vi "ex_getErrorSource.vi"(1 "error in (no error)":errorcluster) -> (0 "error out":errorcluster)   [LabVIEW 2017]
panel:
  in  "Localized ' in ' in message 'foo.vi in bar.vi'":string=" in "
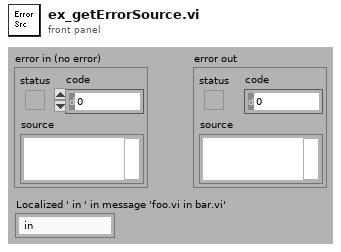
[diagram p1: front panel]
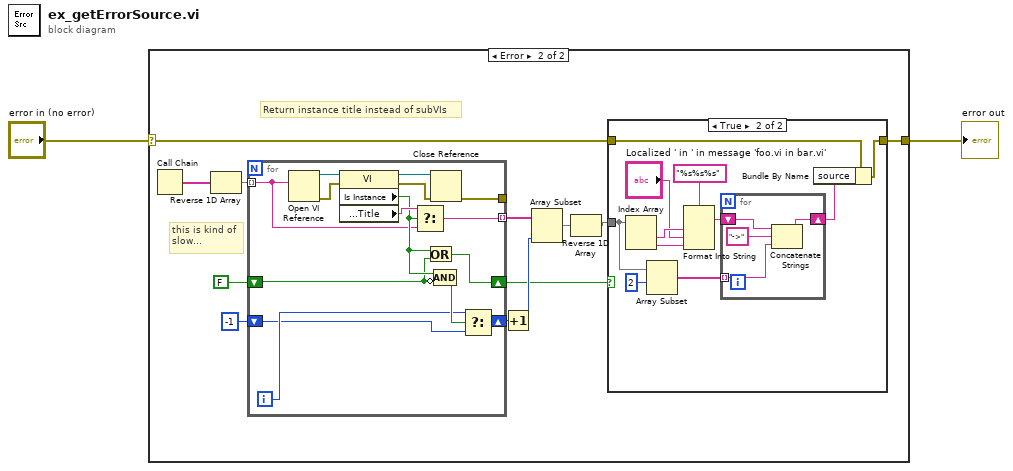
[diagram p0: block diagram]
diagram:
  n1 = case shown="Error" "error in (no error)" {
    selector: "error in (no error)" -> [w3 w5]
    tunnel: [w3 w4] -> w1
    frame No Error {
    }
    frame Error {
      # "this is kind of\nslow..."
      # "Return instance title instead of subVIs"
      n2 = Call Chain() -> (call chain=w15:string[])
      n3 = Reverse 1D Array(array=w15) -> (reversed array=w13:string[])
      n4 = for {
        tunnel: w13 -> [w33] mode=indexing
        tunnel: [w43] -> _
        shift-right: [w38] -> w7
        shift-left: FALSE -> [w39]
        shift-right: [w37] -> w10
        shift-left: -1 -> [w34]
        tunnel: [w32] -> w11 mode=indexing
        i -> [w35]
        n5 = Open VI Reference(vi path=w33) -> (vi reference=w46:refnum<vi>, error out=w44:errorcluster)  [unwired: 1 in, 4 out]
        n6 = property class="VI"(reference=w46, error in=w44) -> (reference out=w42:refnum<vi>, error out=w45:errorcluster, "Is Instance"=w40:bool, "Front Panel Window:Title"=w41:string)
        n7 = Select(t=w41, s=w40, f=w33) -> (s? t:f=w32:string)
        n8 = Or(x=w40, y=w39) -> (x .or. y?=w38:bool)
        n9 = Close Reference(reference=w42, error in (no error)=w45) -> (error out=w43:errorcluster)
        n10 = Compound Arithmetic op=AND(w40, invert w39) -> (w36:bool)
        n11 = Select(t=w35, s=w36, f=w34) -> (s? t:f=w37:i32)
      }
      n12 = Increment(x=w10) -> (x+1=w9:i32)
      n13 = Array Subset(array=w11, length=w9) -> (w8:string[])  [unwired: 1 in]
      n14 = Reverse 1D Array(array=w8) -> (reversed array=w6:string[])
      n15 = case shown="True" w7 {
        tunnel: w6 -> [_ w23]
        tunnel: w5 -> [w16 w26]
        tunnel: [w16 w27] -> w4
        frame False {
        }
        frame True {
          n16 = Index Array(array=w23) -> (element #1=w25:string, element #2=w24:string)  [unwired: 2 in]
          n17 = Array Subset(array=w23, index=2) -> (w21:string[])  [unwired: 1 in]
          n18 = Format Into String(format string="%s%s%s", w25, "Localized ' in ' in message 'foo.vi in bar.vi'", w24) -> (resulting string=w20:string)  [unwired: 2 in, 1 out]
          n19 = for {
            tunnel: w21 -> [w28] mode=indexing
            shift-right: [w31] -> w19
            shift-left: w20 -> [w30]
            n20 = Concatenate Strings(w30, "->" ("string"), w28) -> (w31:string)
          }
          n21 = Bundle By Name(cluster=w26, "source"=w19) -> (w27:errorcluster)
        }
      }
    }
  }
  "error out" <- w1
